vi "Destroy.vi"(8 "error in":errorcluster, 11 "measurement context in":refnum<class "MeasurementContext.lvclass">) -> (0 "error out":errorcluster)   [LabVIEW 2020, in "MeasurementLink Measurement Server.lvlib" / "MeasurementContext.lvclass"]
uses:
  MeasurementContext.lvclass
  MeasurementContext.lvclass/MeasurementContext.ctl
  MeasurementLink gRPC Utilities/gRPC Client Pool/FGV Action.ctl
  MeasurementLink Session Management Client/RPC Messages/ni_measurementlink_sessionmanagement_v1_UnreserveSessionsRequest.ctl
  MeasurementLink gRPC Utilities/gRPC Client Pool/gRPC Client Pool.lvclass
  MeasurementLink Session Management Client/MeasurementLink Session Management Client.lvlib
  MeasurementLink Session Management Client/RPC Messages/nidevice_grpc_Session.ctl
  MeasurementLink Session Management Client/RPC Messages/ni_measurementlink_sessionmanagement_v1_ChannelMapping.ctl
  MeasurementLink Session Management Client/RPC Messages/ni_measurementlink_sessionmanagement_v1_SessionInformation.ctl
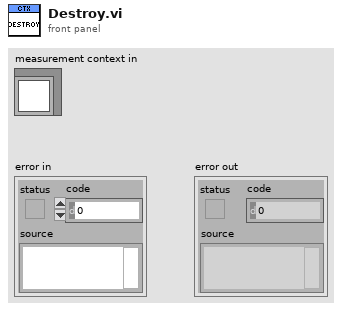
[diagram p1: front panel]
types:
  T1 = typedef "MeasurementLink Session Management Client.lvlib/ni_measurementlink_sessionmanagement_v1_UnreserveSessionsRequest.ctl" = cluster{"sessions":T2[]}
  T2 = typedef "MeasurementLink Session Management Client.lvlib/ni_measurementlink_sessionmanagement_v1_SessionInformation.ctl" = cluster{"session":T3, "resource_name":string, "channel_list":string, "instrument_type_id":string, "session_exists":bool, "channel_mappings":T4[]}
  T3 = typedef "MeasurementLink Session Management Client.lvlib/nidevice_grpc_Session.ctl" = cluster{"name":string}
  T4 = typedef "MeasurementLink Session Management Client.lvlib/ni_measurementlink_sessionmanagement_v1_ChannelMapping.ctl" = cluster{"pin_or_relay_name":string, "site":i32, "channel":string}
  T5 = typedef "MeasurementLink gRPC Utilities.lvlib/gRPC Client Pool.lvclass/FGV Action.ctl" = enum16{"Get Discovery Client", "Get Session Client", "Get Pinmap Client", "Destroy Clients"}
  T6 = typedef "MeasurementLink Measurement Server.lvlib/MeasurementContext.lvclass/Data.ctl" = cluster{"PinMapContext":T7, "gRPCServerId":T8, "IMeasurementService":refnum<class "IMeasurementService.lvclass">, "MeasurementPluginService":refnum<class "MeasurementPluginService.lvclass">, "session infos to unreserve":map{refnum<class "Session Reservation.lvclass">, T2[]}}
  T7 = typedef "MeasurementLink Measurement Server.lvlib/PinMapContext.ctl" = cluster{"pin_map_id":string, "sites":i32[]}
  T8 = typedef "grpc-lvsupport-release.lvlib/grpcId.ctl" = u64
  T9 = map{refnum<class "Session Reservation.lvclass">, T2[]}
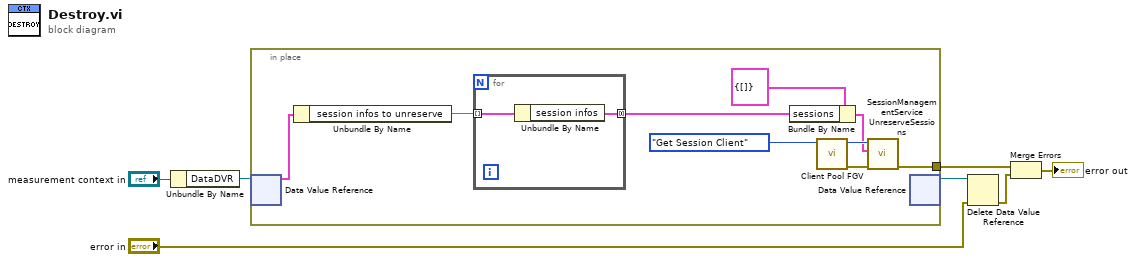
[diagram p0: block diagram]
diagram:
  n1 = Unbundle By Name("measurement context in") -> ("DataDVR"=w6:refnum<data-value>)
  n2 = in-place {
    in-place-border: [w10] -> w4
    n3 = in-place-dvr #1(w6) -> (w16:T6)  [unwired: 1 out]
    n4 = Unbundle By Name(w16) -> ("session infos to unreserve"=w9:T9)
    n5 = for {
      tunnel: w9 -> [w18] mode=indexing
      tunnel: [w17] -> w8 mode=concatenating
      n6 = Unbundle By Name(w18) -> ("session infos"=w17:T2[])
    }
    n7 = Bundle By Name(cluster=T1 {"sessions"=[]} ("Request Data"), "sessions"=w8) -> (w12:T1)
    n8 = call "Client Pool FGV.vi"("Action"=FGV_Action."Get Session Client") -> ("error out"=w11:errorcluster, "grpc client id"=w14:T8)  [unwired: 9 in]
    n9 = call "SessionManagementService UnreserveSessions.vi"("error in"=w11, "Request Data"=w12, "gRPC ID"=w14) -> ("error out"=w10:errorcluster)  [unwired: 6 in, 2 out]
    n10 = in-place-dvr #1() -> (w5:refnum<data-value>)  [unwired: 1 in, 1 out]
  }
  n11 = Delete Data Value Reference(data value reference=w5, error in="error in") -> (error out=w1:errorcluster)  [unwired: 1 out]
  n12 = Merge Errors(w4, w1) -> (→"error out":errorcluster)
